vi "Tx and Rx Streaming (Host).vi"() -> ()   [LabVIEW 2018]
doc: "This template is for the Simple NI-USRP Streaming design, a design that shows the basics of streaming data to and from an NI USRP-294x/295x device. Refer to the block diagram for more information about how to use this template."
uses:
  <vilib>/userdefined/Silver/nirio_resource_slv.ctl
  SubVIs/Start Trigger.ctl
  <vilib>/Utility/error.llb/DialogType.ctl
panel:
  in  "config tab":enum32{"Tx Configuration", "Rx Configuration"}(tab)
  in  "tx config":T2={"rf enable 0"=TRUE, "rf config 0"={"antenna"="TX1", "frequency"=2000000000.0, "lo frequency"=-1.0, "level"=0.0}, "rf enable 1"=TRUE, "rf config 1"={"antenna"="TX1", "frequency"=2000000000.0, "lo frequency"=-1.0, "level"=0.0}, "transfer mode"=enum."Finite", "sample rate"=10000000.0, "number of samples"=8192, "start trigger"=enum."Immediate", "tone frequency"=100000.0} {"tone frequency" format="%#.3pHz"; "sample rate" format="%#.3pS/s"; "rf config 0"."level" format="%#_gdBm"; "rf config 0"."lo frequency" format="%#.3pHz"; "rf config 0"."frequency" format="%#.3pHz"; "rf config 1"."level" format="%#_gdBm"; "rf config 1"."lo frequency" format="%#.3pHz"; "rf config 1"."frequency" format="%#.3pHz"}
  in  "rx config":T3={"rf enable 0"=TRUE, "rf config 0"={"antenna"="RX2", "frequency"=2000000000.0, "lo frequency"=-1.0, "level"=0.0}, "rf enable 1"=TRUE, "rf config 1"={"antenna"="RX2", "frequency"=2000000000.0, "lo frequency"=-1.0, "level"=0.0}, "transfer mode"=enum."Finite", "sample rate"=10000000.0, "number of samples"=8192, "start trigger"=enum."Immediate"} {"sample rate" format="%#.3pS/s"; "rf config 1"."level" format="%#_gdBm"; "rf config 1"."lo frequency" format="%#.3pHz"; "rf config 1"."frequency" format="%#.3pHz"; "rf config 0"."level" format="%#_gdBm"; "rf config 0"."lo frequency" format="%#.3pHz"; "rf config 0"."frequency" format="%#.3pHz"}
  out "acquiring":bool caption="Acquiring"
  in  "tx.stop":bool
  out "generating":bool caption="Generating"
  in  "USRP RIO device":T4="RIO0" caption="USRP RIO Device"
  in  "reference frequency source":string(combo)="Internal" caption="Reference Frequency Source"
  in  "indicator tab":T5(tab)
  out "tx.output waveform":waveform(dbl)[](graph) caption="Output Waveform"
  out "power spectrum":cluster{"f0":dbl, "df":dbl, "magnitude":dbl[]}[](graph) caption="Power Spectrum"
  out "power level":dbl[][](graph) caption="Power Level"
  out "iq data":waveform(dbl)[](graph) caption="I & Q Data"
  out "rx.coerced config":T6 caption="Rx" {"coerced sample rates" format="%#.3pS/s"; "coerced levels" format="%#.3gdBm"; "coerced lo frequencies" format="%#.3pHz"; "coerced frequencies" format="%#.3pHz"}
  out "tx.coerced config":T6 caption="Tx" {"coerced sample rates" format="%#.3pS/s"; "coerced levels" format="%#.3gdBm"; "coerced lo frequencies" format="%#.3pHz"; "coerced frequencies" format="%#.3pHz"}
  in  "rx.stop":bool
  # "This template is for the Simple NI-USRP Streaming design, a design that shows the basics of streaming data on a USRP RIO device. See the block diagram for more information on how to use this template."
  # "Simple Tx and Rx Streaming"
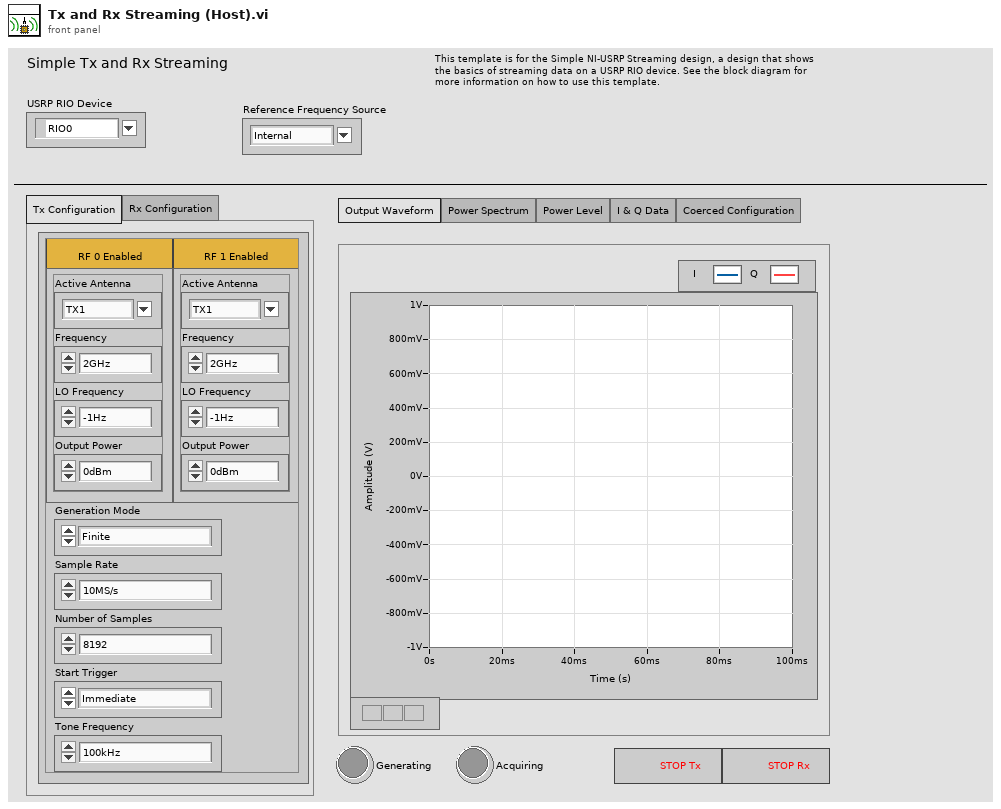
[diagram p1: front panel]
types:
  T1 = typedef "Start Trigger.ctl" = enum8{"Software", "Digital Edge", "Rx Start Trigger", "Tx Start Trigger", "Immediate", "Future Time Event"}
  T2 = cluster{"rf enable 0":bool, "rf config 0":cluster{"antenna":string, "frequency":dbl, "lo frequency":dbl, "level":dbl}, "rf enable 1":bool, "rf config 1":cluster{"antenna":string, "frequency":dbl, "lo frequency":dbl, "level":dbl}, "transfer mode":enum16{"Finite", "Continuous"}, "sample rate":dbl, "number of samples":u32, "start trigger":T1, "tone frequency":dbl}
  T3 = cluster{"rf enable 0":bool, "rf config 0":cluster{"antenna":string, "frequency":dbl, "lo frequency":dbl, "level":dbl}, "rf enable 1":bool, "rf config 1":cluster{"antenna":string, "frequency":dbl, "lo frequency":dbl, "level":dbl}, "transfer mode":enum16{"Finite", "Continuous"}, "sample rate":dbl, "number of samples":u32, "start trigger":T1}
  T4 = typedef "nirio_resource_slv.ctl" = tag
  T5 = enum32{"Output Waveform", "Power Spectrum", "Power Level", "I & Q Data", "Coerced Configuration"}
  T6 = cluster{"coerced frequencies":dbl[], "coerced lo frequencies":dbl[], "coerced levels":dbl[], "coerced sample rates":dbl[]}
  T7 = typedef "DialogType.ctl" = u16
  T8 = typedef "Rx Channels.ctl" = cluster{"rx config":cluster{"channel configuration":cluster{"channel enable":bool, "channel configuration":cluster{"antenna":string, "frequency":dbl, "lo frequency":dbl, "level":dbl}}[], "transfer mode":enum16{"Finite", "Continuous"}, "sample rate":dbl, "number of samples":u32, "start trigger":T1}, "reference frequency source":string, "rx.data sink":enum16{"SFP Port 0", "SFP Port 1", "Host"}, "rx.enabled channels":string[], "vertical range":dbl[], "rx.coerced configurations":cluster{"coerced frequencies":dbl[], "coerced lo frequencies":dbl[], "coerced levels":dbl[], "coerced sample rates":dbl[]}}
  T9 = typedef "Tx Channels.ctl" = cluster{"tx config":cluster{"channel configuration":cluster{"channel enable":bool, "channel configuration":cluster{"antenna":string, "frequency":dbl, "lo frequency":dbl, "level":dbl}}[], "transfer mode":enum16{"Finite", "Continuous"}, "sample rate":dbl, "number of samples":u32, "start trigger":T1, "tone frequency":dbl}, "reference frequency source":string, "tx.data source":enum16{"SFP Port 0", "SFP Port 1", "Host"}, "tx.enabled channels":string[], "I":i16[], "Q":i16[], "tx.coerced configurations":cluster{"coerced frequencies":dbl[], "coerced lo frequencies":dbl[], "coerced levels":dbl[], "coerced sample rates":dbl[]}}
  T10 = typedef "niUsrpRio Config v1 Host.lvlib/niUsrpRio Session.ctl" = cluster{"FPGA Interface":refnum<k20>, "RIO Interface Number":u32, "Data Clock Rate":u32, "FPGA Data Clock Rate":u32, "Global Settings Register Bus":T11, "Radio 0 Settings Register Bus":T11, "Radio 1 Settings Register Bus":T11, "Radio Settings Bus Semaphore":T12, "DB Queues":T13[], "Characterization Data Valid?":bool, "EEPROM Header":T14, "Device Data Header":T15, "EEPROM Characterization Header":T16, "Characterization Data":T17[], "FPGA Current Version":u32, "FPGA Oldest Compatible Version":u32, "Fixed Logic Current Version":u32, "Fixed Logic Oldest Compatible Version":u32, "FPGA Radio Settings Bus Current Version":u32, "FPGA Radio Settings Bus Oldest Compatible Version":u32, "FPGA Board Config Current Version":u32, "FPGA Board Config Oldest Compatible Version":u32, "Daughterboard Clock Rate":u32, "daughterboard configuration session handles":u64[]}
  T11 = typedef "niInstr Register Bus v0 Host.lvlib/Register Bus Session.ctl" = refnum<queue>
  T12 = typedef "Semaphore RefNum" = refnum<k1>
  T13 = typedef "niUsrpRio Config v1 Host.lvlib/DB Queue Reference.ctl" = refnum<queue>
  T14 = typedef "niUsrpRio Config v1 Host.lvlib/EEPROM Header.ctl" = cluster{"Checksum":u32, "Product Code":u16, "Hardware Current Version":u16, "Hardware Oldest Compatible Version":u16, "EEPROM Map Current Version":u16, "EEPROM Map Oldest Compatible Version":u16, "User Password":string, "Pointer to Factory Header":u32, "Pointer to User Header":u32, "Recommended Interval":u16, "Number of Reserved Bytes":i32, "Number of Daughterboards":u8, "Daughterboard IDs":u16[], "Daughterboard Serial Numbers":string[]}
  T15 = typedef "niUsrpRio Config v1 Host.lvlib/EEPROM Device Data Header.ctl" = cluster{"Checksum":u32, "Number of Channels":u8, "Number of Gain Settings":u16[], "Pointer to Characterization Data":u32[], "Number of Reserved Bytes":i32, "Number of Frequencies":u16[]}
  T16 = typedef "niUsrpRio Config v1 Host.lvlib/EEPROM Characterization Header.ctl" = cluster{"Checksum":u32, "Date":timestamp, "Temperature":sgl, "Misc. Info":string, "Pointer to Device Data Header":u32, "Number of Reserved Bytes":i32}
  T17 = typedef "niUsrpRio Config v1 Host.lvlib/Characterization Data.ctl" = cluster{"Gains[dB]":dbl[], "Frequencies [Hz]":dbl[], "IQ Imbalance Table":T18[], "Measured Gains[dB]":dbl[][]}
  T18 = typedef "niUsrpRio Config v1 Host.lvlib/IQ Imbalance.ctl" = cluster{"Gain Imbalance [linear]":dbl, "Phase Imbalance [radians]":dbl, "Offset":cdb}
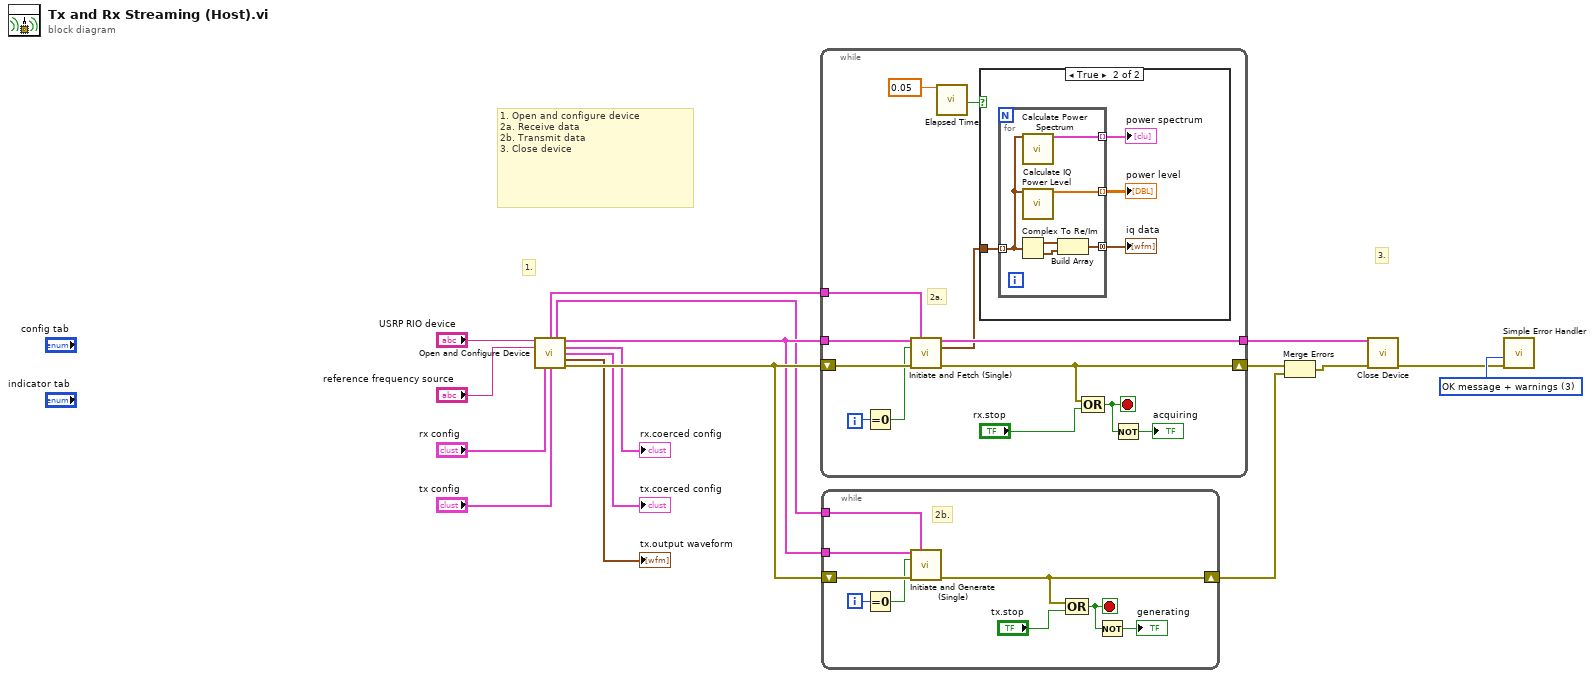
[diagram p0: block diagram]
diagram:
  w16 = T7 3 items=["no dialog", "OK message", "continue or stop message", "OK message + warnings", "continue/stop + warnings"] ("type of dialog (OK msg:1)")
  # "3."
  # "1. Open and configure device\n2a. Receive data\n2b. Transmit data\n3. Close device"
  # "1."
  n1 = call "Open and Configure Device.vi"("USRP RIO Device"="USRP RIO device", "reference frequency source"="reference frequency source", "rx config"="rx config", "tx config"="tx config") -> ("rx channels"=w14:T8, "tx channels"=w1:T9, "niUsrpRio Session (out)"=w2:T10, "rx.coerced configurations"=→"rx.coerced config":T6, "tx.coerced configurations"=→"tx.coerced config":T6, "tx.output waveform"=→"tx.output waveform":waveform(dbl)[], "error out"=w17:errorcluster)  [unwired: 5 in]
  n2 = while {
    tunnel: w2 -> [w28]
    tunnel: [w25] -> w5
    tunnel: w14 -> [w22]
    shift-right: [w26] -> w6
    shift-left: w17 -> [w29]
    i -> [w27]
    stop <- w23 stop-if-true
    # "2a."
    # "Acquire and Fetch a waveform"
    n3 = Equal To 0?(x=w27) -> (x = 0?=w18:bool)
    n4 = call "Initiate and Fetch (Single).vi"("niUsrpRio Session"=w28, "rx channels"=w22, "first iteration"=w18, "error in"=w29) -> ("niUsrpRio Session (out)"=w25:T10, "complex baseband data"=w19:waveform(cdb)[], "error out"=w26:errorcluster)  [unwired: 9 in]
    n5 = call "Elapsed Time"("Time Target (s)"=0.05 ("retrigger delay")) -> ("Time has Elapsed"=w21:bool)  [unwired: 11 in, 7 out]
    n6 = case shown="TRUE" w21 {
      tunnel: w19 -> [_ w34]
      frame False {
      }
      frame True {
        n7 = for {
          tunnel: [w38] -> w33 mode=concatenating
          tunnel: [w37] -> w32 mode=indexing
          tunnel: [w36] -> w31 mode=indexing
          tunnel: w34 -> [w35] mode=indexing
          n8 = Complex To Re/Im(x + iy=w35) -> (x=w40:waveform(dbl), y=w39:waveform(dbl))
          n9 = call "Calculate Power Spectrum.vi"("waveform"=w35) -> ("power spectrum (dBm)"=w36:cluster{"f0":dbl, "df":dbl, "magnitude":dbl[]})  [unwired: 14 in]
          n10 = call "Calculate IQ Power Level.vi"("iq data"=w35) -> ("power level (dBm)"=w37:dbl[])  [unwired: 14 in]
          n11 = Build Array(w40, w39) -> (w38:waveform(dbl)[])
        }
        "power level" <- w32
        "power spectrum" <- w31
        "iq data" <- w33
      }
    }
    n12 = Compound Arithmetic op=OR(w26, "rx.stop") -> (w23:bool)
    n13 = Not(x=w23) -> (.not. x?=→"acquiring":bool)
  }
  n14 = while {
    tunnel: w2 -> [w47]
    tunnel: w1 -> [w42]
    shift-right: [w45] -> w7
    shift-left: w17 -> [w46]
    i -> [w44]
    stop <- w43 stop-if-true
    # "2b."
    # "Acquire and Fetch a waveform"
    n15 = Equal To 0?(x=w44) -> (x = 0?=w41:bool)
    n16 = call "Initiate and Generate (Single).vi"("niUsrpRio Session"=w47, "tx channels"=w42, "first iteration"=w41, "error in"=w46) -> ("error out"=w45:errorcluster)  [unwired: 10 in, 1 out]
    n17 = Compound Arithmetic op=OR(w45, "tx.stop") -> (w43:bool)
    n18 = Not(x=w43) -> (.not. x?=→"generating":bool)
  }
  n19 = Merge Errors(w6, w7) -> (w13:errorcluster)
  n20 = call "Close Device.vi"("niUsrpRio Session"=w5, "error in"=w13) -> ("error out"=w15:errorcluster)  [unwired: 13 in]
  n21 = call <vilib>:"Simple Error Handler.vi"("type of dialog (OK msg:1)"=w16, "error in (no error)"=w15) -> ()  [unwired: 3 in, 5 out]
